vi "Initialize System Actors.vi"(8 "error in (no error)":errorcluster, 10 "Root Actor In":refnum<class "Root Actor.lvclass">, 11 "System Modules Factory in":refnum<class "System Modules Factory.lvclass">) -> (0 "error out":errorcluster, 2 "Root Actor Out":refnum<class "Root Actor.lvclass">, 3 "System Modules Factory out":refnum<class "System Modules Factory.lvclass">)   [LabVIEW 2024, in "System Modules Factory.lvclass"]
uses:
  System Modules Factory.lvclass
  Actor/Root Actor/Root Actor.lvclass
  System Modules Factory.lvclass/System Modules Factory.ctl
  Actor/Root Actor/Root Actor.lvclass/Root Actor.ctl
  Actor/System Actor/System Actor.lvclass/System Actor.ctl
  Actor/System Actor/Public Data/Write Self Messenger Location.vi
  Actor/Root Actor/Public Data/Read Node Controller.vi
  Actor/Root Actor/Public Data/Write Node Controller.vi
  Actor Assistant/Root Actor Node Controller/Node Controller.lvclass
  Actor/System Actor/System Actor.lvclass
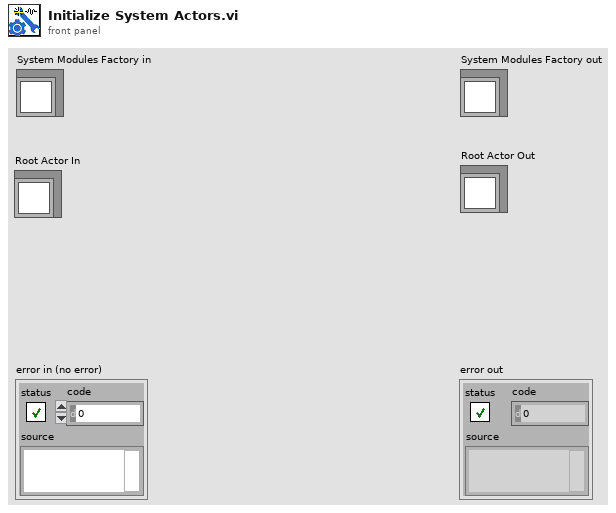
[diagram p1: front panel]
types:
  T1 = typedef "Config Parameters.ctl" = cluster{"Actors":refnum<class "System Actor.lvclass">[], "Rendevous Treads":i32[], "Actors Address":refnum<class "Mail Strategy.lvclass">[], "Root Actor Address":refnum<class "Mail Strategy.lvclass">}
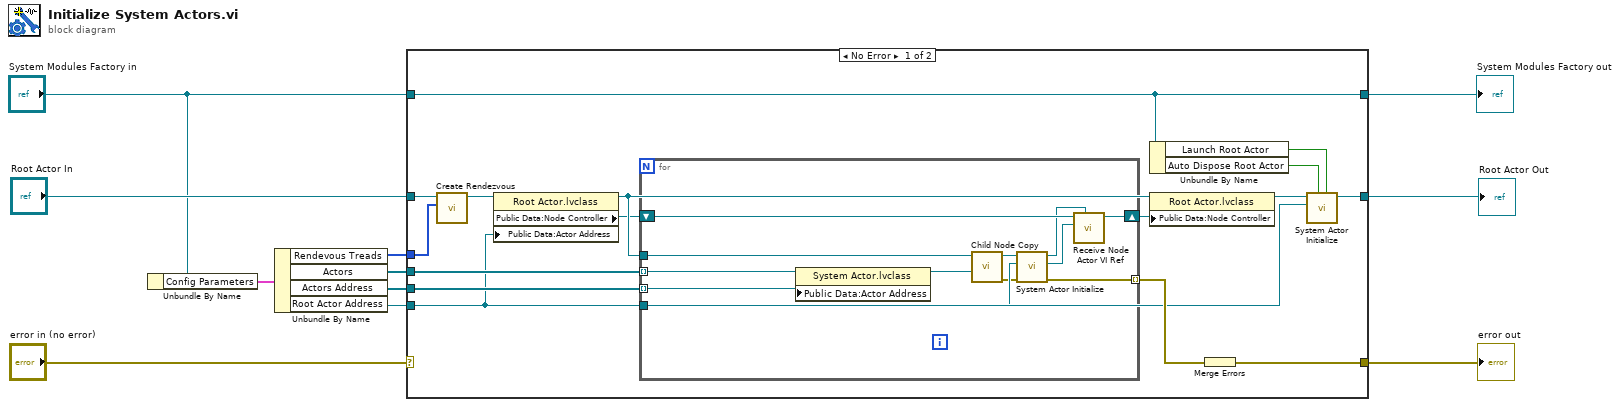
[diagram p0: block diagram]
diagram:
  n1 = Unbundle By Name("System Modules Factory in") -> ("Config Parameters"=w2:T1)
  n2 = Unbundle By Name(w2) -> ("Rendevous Treads"=w8:i32[], "Actors"=w10:refnum<class "System Actor.lvclass">[], "Actors Address"=w9:refnum<class "Mail Strategy.lvclass">[], "Root Actor Address"=w7:refnum<class "Mail Strategy.lvclass">)
  n3 = case shown="No Error" "error in (no error)" {
    selector: "error in (no error)" -> [_ w42]
    tunnel: [w22 w42] -> w4
    tunnel: [w15 w41] -> w6
    tunnel: "System Modules Factory in" -> [w15 w41]
    tunnel: "Root Actor In" -> [w26 w40]
    tunnel: w10 -> [w27 _]
    tunnel: w9 -> [w25 _]
    tunnel: w8 -> [w24 _]
    tunnel: w7 -> [w12 _]
    tunnel: [w16 w40] -> w1
    frame No Error {
      n4 = call "Create Rendezvous.vi"("Treads"=w24, "Actor In"=w26) -> ("Actor Out"=w21:refnum<class "Root Actor.lvclass">)  [unwired: 8 in, 1 out]
      n5 = property class="Root Actor.lvclass"(reference=w21, "Public Data:Actor Address"=w12) -> (reference out=w20:refnum<class "Root Actor.lvclass">, "Public Data:Node Controller"=w19:refnum<class "Node Controller.lvclass">)  [unwired: 1 in, 1 out]
      n6 = for {
        tunnel: w20 -> [w39]
        tunnel: w27 -> [w38] mode=indexing
        tunnel: w25 -> [w37] mode=indexing
        tunnel: w12 -> [w36]
        tunnel: [w32] -> w23 mode=indexing
        shift-right: [w30] -> w18
        shift-left: w19 -> [w31]
        n7 = property class="System Actor.lvclass"(reference=w38, "Public Data:Actor Address"=w37) -> (reference out=w33:refnum<class "System Actor.lvclass">)  [unwired: 1 in, 1 out]
        n8 = call-dynamic "Child Node Copy.vi"("Child In"=w33, "Ancestor In"=w39) -> ("error out"=w34:errorcluster, "Child Out"=w35:refnum<class "System Actor.lvclass">)  [unwired: 8 in]
        n9 = call-dynamic "System Actor Initialize.vi"("error in (no error)"=w34, "Root Actor Address"=w36, "System Actor in"=w35) -> ("error out"=w32:errorcluster, "VI Refnum"=w29:refnum<vi>, "System Actor out"=w28:refnum<class "System Actor.lvclass">)  [unwired: 6 in]
        n10 = call-dynamic "Receive Node Actor VI Ref.vi"("System Actor In"=w28, "VI Refnum In"=w29, "Node Controller in"=w31) -> ("Node Controller out"=w30:refnum<class "Node Controller.lvclass">)  [unwired: 6 in, 2 out]
      }
      n11 = Unbundle By Name(w15) -> ("Launch Root Actor"=w14:bool, "Auto Dispose Root Actor"=w13:bool)
      n12 = property class="Root Actor.lvclass"(reference=w20, "Public Data:Node Controller"=w18) -> (reference out=w17:refnum<class "Root Actor.lvclass">)  [unwired: 1 in, 1 out]
      n13 = Merge Errors(w23) -> (w22:errorcluster)
      n14 = call-dynamic "System Actor Initialize.vi"("Launching"=w14, "Auto Dispose Ref"=w13, "Root Actor Address"=w12, "System Actor in"=w17) -> ("System Actor out"=w16:refnum<class "Root Actor.lvclass">)  [unwired: 5 in, 2 out]
    }
    frame Error {
    }
  }
  "error out" <- w4
  "System Modules Factory out" <- w6
  "Root Actor Out" <- w1
